vi "main.vi"(11 "Module Admin":refnum<class "Delacor_lib_QMH_Module Admin.lvclass">) -> ()   [LabVIEW 2020, in "G-AI Core.lvlib"]
doc: "This template is based off of the Queued Message Handler design pattern and the Queued Message Handler project template that ships with LabVIEW.\n\nThe main difference is that the queue is private to this module and communication between modules is performed via Broadcast and Request events.\n\nRequest events are wrapped in public API methods and are handled in the Event Handling Loop (EHL) of this VI. Any module can register for Broadcast events sent by this module. The EHL generates messages based on user interface actions.\n\nThe Message Handling Loop (MHL) processes messages generated by the EHL, or by other messages. The messages are string values, so new messages can be added easily to the Message Cases case structure in the MHL. Each message cluster can also provide an optional value for Message Data, which is a variant that can be converted to whatever message-specific data is required.\n_____\nBased on DQMH Dev Tools: Project Template 7.1.2.1547."
uses:
  G-AI Core.lvlib
  <vilib>/Delacor/Delacor QMH/Libraries/Module Admin_class/Delacor_lib_QMH_Module Admin.lvclass
  Module Data--cluster.ctl
  <vilib>/Delacor/Delacor QMH/Libraries/Message Queue_class/Delacor_lib_QMH_Message Queue.lvclass/Delacor_lib_QMH_Message Queue.ctl
  Stop Argument--cluster.ctl
  <vilib>/Delacor/Delacor QMH/Libraries/Module Admin_class/Delacor_lib_QMH_Module Admin.lvclass/Delacor_lib_QMH_Module Admin.ctl
  Store Reference Argument--cluster.ctl
  Store Reference (Reply Payload)--cluster.ctl
  Get Reference Argument--cluster.ctl
  Get Reference (Reply Payload)--cluster.ctl
  New VI Argument--cluster.ctl
  New VI (Reply Payload)--cluster.ctl
  Open VI Reference Argument--cluster.ctl
  Open VI Reference (Reply Payload)--cluster.ctl
  <vilib>/Utility/miscctls.llb/LVPointTypeDef.ctl
  <vilib>/Delacor/Delacor QMH/Libraries/Message Queue_class/Delacor_lib_QMH_Enqueue Message (Single).vi
  <vilib>/Delacor/Delacor QMH/Libraries/Module Admin_class/Delacor_lib_QMH_Get External Launch.vi
  <vilib>/Delacor/Delacor QMH/Libraries/Message Queue_class/Delacor_lib_QMH_Message Queue.lvclass
  <vilib>/jgoebel/LabVIEW MCP Server SDK/src/MCP Server/jg_mcp_MCP Server.lvlib
panel:
  out "Log":string
  out "error out":errorcluster
  out "Status":string
  in  "Simulate MHL Error":bool
  in  "Simulate EHL Error":bool
  # "Keep this VI open to make the G-AI MCP-Server reachable from your\nMCP Client (e.g. Claude Desktop).\nAdd MCP Server to mcp_config.json or claude_desktop_config.json"
  # "Server Name: G-AI\nServer Port: 36987\nServer URL: /mcp/server"
  # "https://github.com/JanGoebel/G-AI"
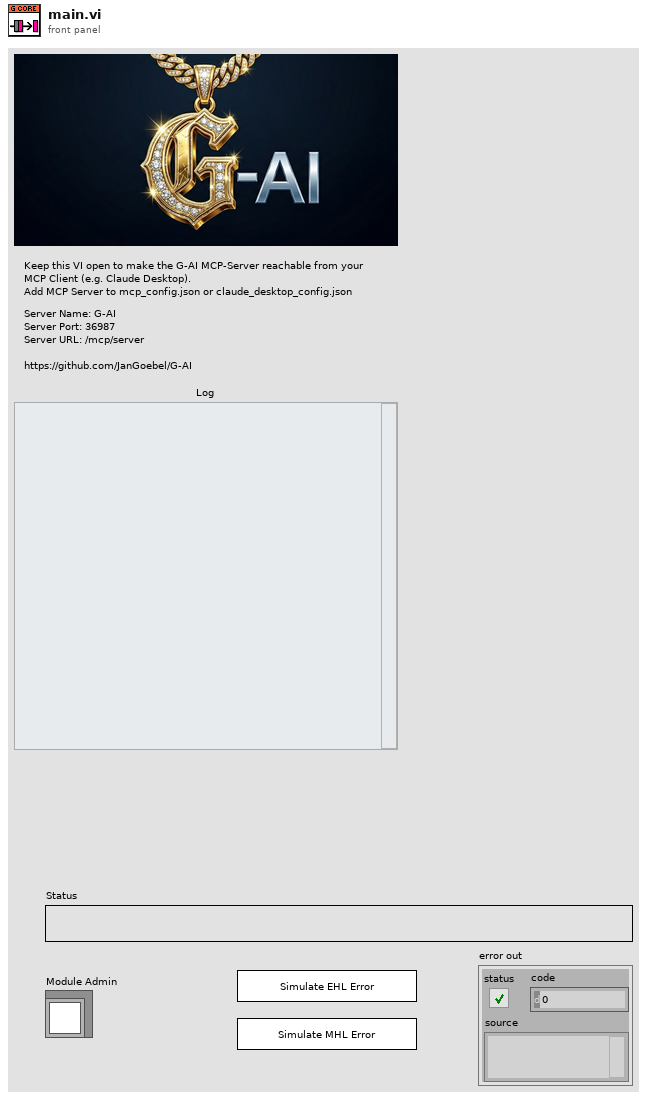
[diagram p1: front panel]
types:
  T1 = typedef "G-AI Core.lvlib/Module Data--cluster.ctl" = cluster{"Status":string, "LookupTable":variant, "last id":i32, "MCP reference":i32}
  T2 = typedef "G-AI Core.lvlib/Request Events--cluster.ctl" = cluster{"Stop Module":refnum<user-event>, "Show Panel":refnum<user-event>, "Hide Panel":refnum<user-event>, "Get Module Execution Status":refnum<user-event>, "Show Diagram":refnum<user-event>, "Store Reference":refnum<user-event>, "Get Reference":refnum<user-event>, "New VI":refnum<user-event>, "Open VI Reference":refnum<user-event>}
  T3 = typedef "jg_mcp_MCP Server.lvlib/jg_mcp_User Events.ctl" = cluster{"onError":refnum<user-event>, "onRpc":refnum<user-event>}
  T4 = enum32{"invalid lock state", "Not Locked", "Locked (No Password)", "Password-protected"}
  T5 = typedef "G-AI Core.lvlib/Stop Argument--cluster.ctl" = cluster{"Origin":string, "Exit via Stop Module Req?":bool, "Wait for Module to stop?":bool}
  T6 = typedef "G-AI Core.lvlib/Store Reference Argument--cluster.ctl" = cluster{"Reference":variant, "Wait Notifier":refnum<notifier>, "wait for reply":bool}
  T7 = typedef "G-AI Core.lvlib/Get Reference Argument--cluster.ctl" = cluster{"id":string, "Wait Notifier":refnum<notifier>, "wait for reply":bool}
  T8 = typedef "G-AI Core.lvlib/New VI Argument--cluster.ctl" = cluster{"Wait Notifier":refnum<notifier>, "wait for reply":bool}
  T9 = typedef "G-AI Core.lvlib/Open VI Reference Argument--cluster.ctl" = cluster{"VI Path":string, "options":i32, "password":string, "Wait Notifier":refnum<notifier>, "wait for reply":bool}
  T10 = typedef "LVPointTypeDef.ctl" = cluster{"Horizontal":i16, "Vertical":i16}
  T11 = enum32{"Invalid", "Standard", "Closed", "Hidden", "Minimized", "Maximized"}
  T12 = typedef "G-AI Core.lvlib/New VI (Reply Payload)--cluster.ctl" = cluster{"VI Refnum":refnum<vi>, "error":errorcluster}
  T13 = typedef "G-AI Core.lvlib/Open VI Reference (Reply Payload)--cluster.ctl" = cluster{"VI Refnum":refnum<vi>, "error":errorcluster}
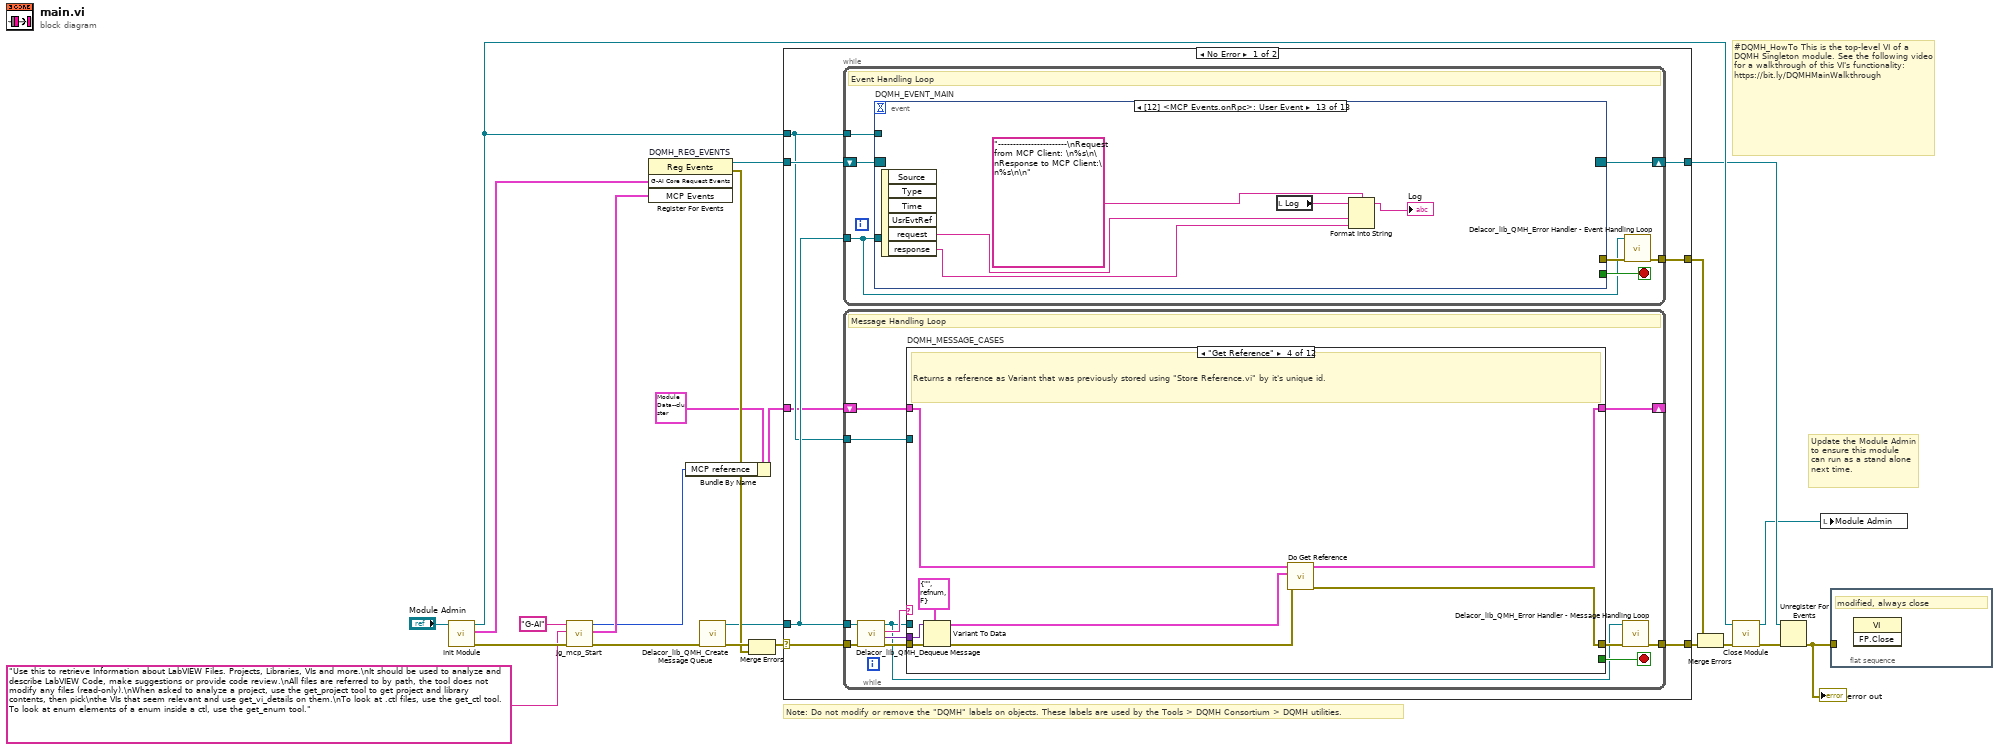
[diagram p0: block diagram]
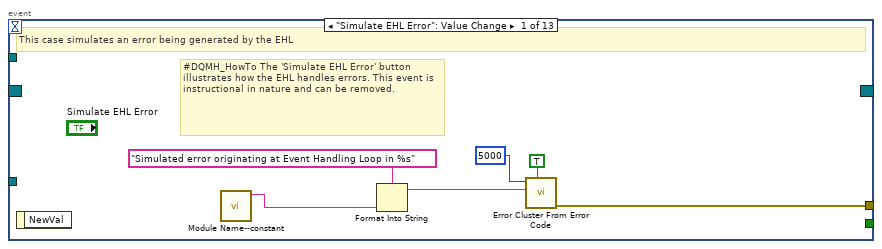
[diagram p2: hidden frame]
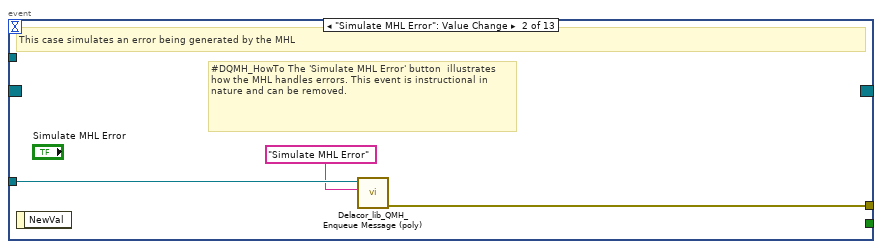
[diagram p3: hidden frame]
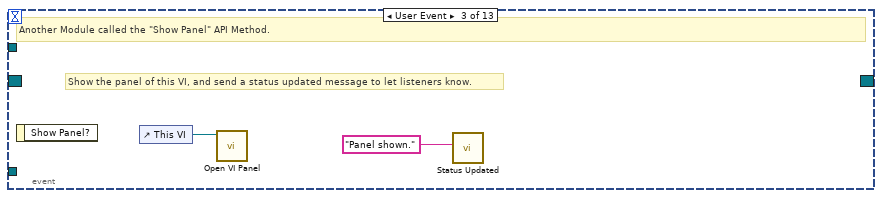
[diagram p4: hidden frame]
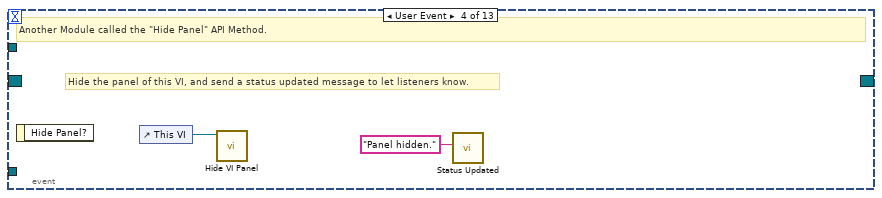
[diagram p5: hidden frame]
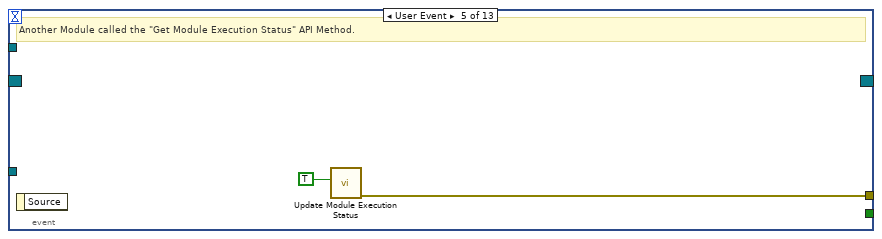
[diagram p6: hidden frame]
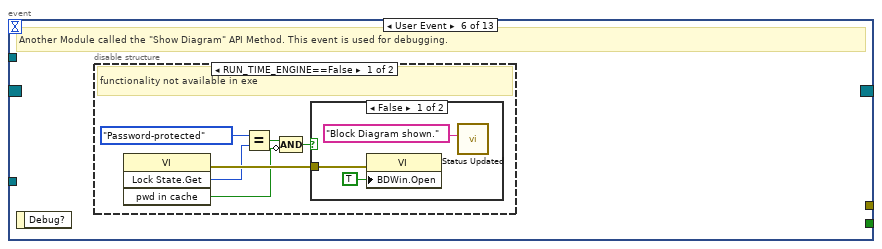
[diagram p7: hidden frame]
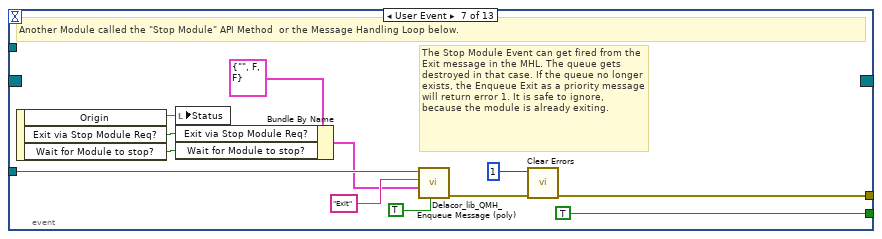
[diagram p10: hidden frame]
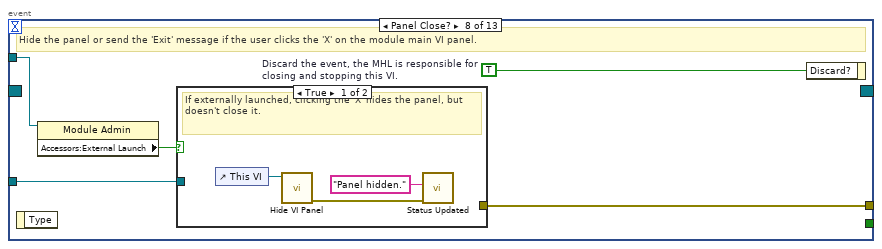
[diagram p11: hidden frame]
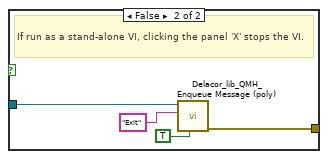
[diagram p12: hidden frame]
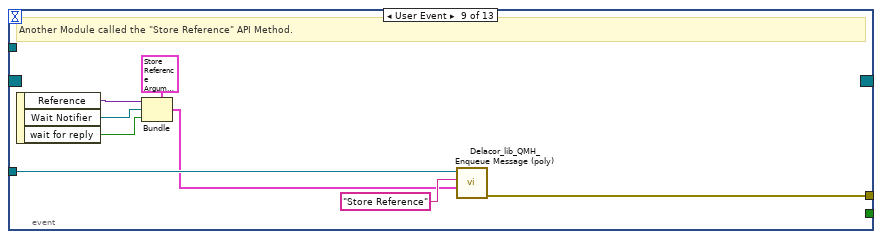
[diagram p13: hidden frame]
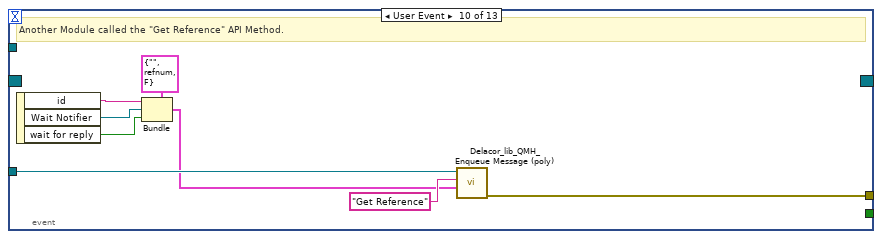
[diagram p14: hidden frame]
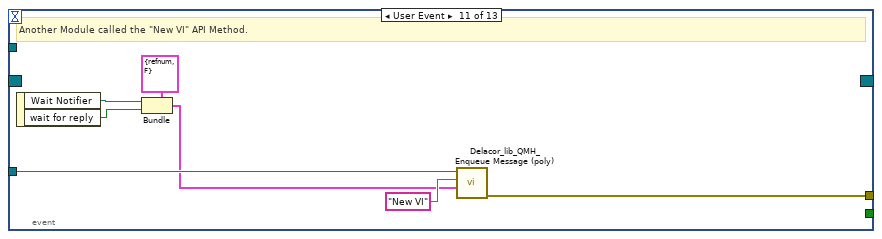
[diagram p15: hidden frame]
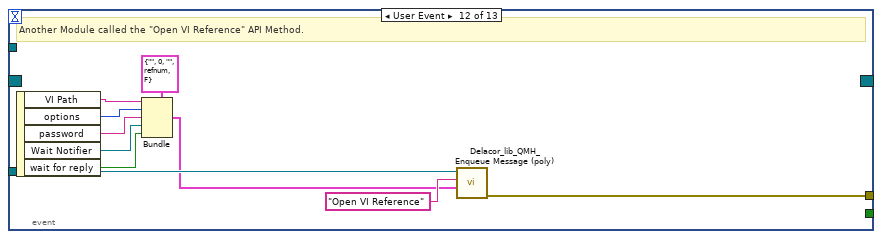
[diagram p16: hidden frame]
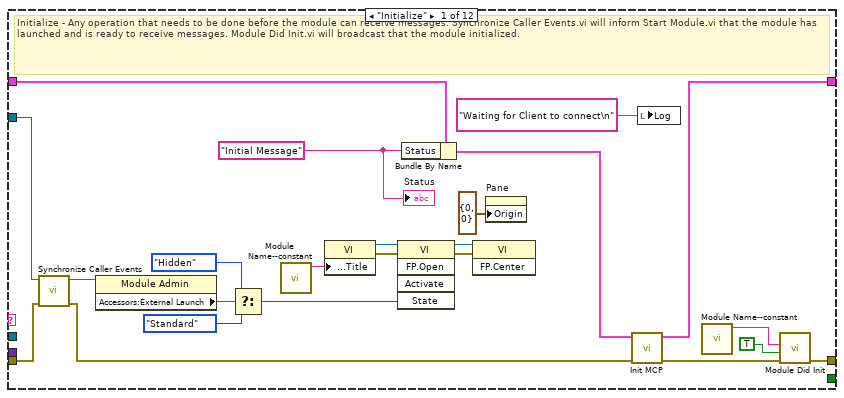
[diagram p17: hidden frame]
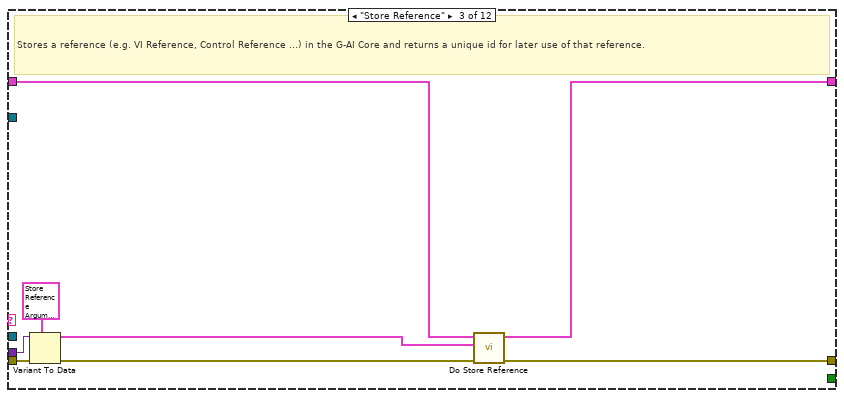
[diagram p19: hidden frame]
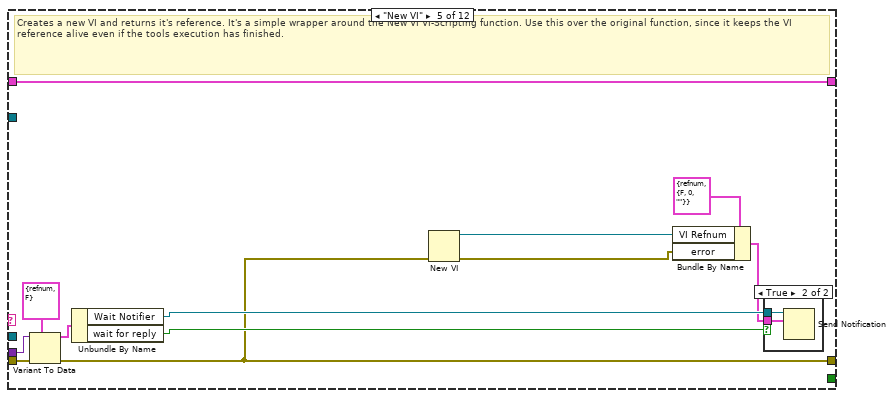
[diagram p20: hidden frame]
diagram:
  # "#DQMH_HowTo This is the top-level VI of a DQMH Singleton module. See the following video for a walkthrough of this VI's functionality: https://bit.ly/DQMHMainWalkthrough"
  # "Note: Do not modify or remove the \"DQMH\" labels on objects. These labels are used by the Tools > DQMH Consortium > DQMH utilities."
  # "Update the Module Admin to ensure this module can run as a stand alone next time."
  n1 = call "Init Module.vi"("Singleton Module Admin in"="Module Admin") -> ("error out"=w9:errorcluster, "G-AI Core Request Events"=w13:T2, "Singleton Module Admin out"=w16:refnum<class "Delacor_lib_QMH_Module Admin.lvclass">)  [unwired: 8 in]
  n2 = call <vilib>:"jg_mcp_Start.vi"("error in (no error)"=w9, "Description"="Use this to retrieve Information about LabVIEW Files. Projects, Libraries, VIs and more.\nIt should be used to analyze and describe LabVIEW Code, make suggestions or provide code review.\nAll files are referred to by path, the tool does not modify any files (read-only).\nWhen asked to analyze a project, use the get_project tool to get project and library contents, then pick\nthe VIs that seem relevant and use get_vi_details on them.\nTo look at .ctl files, use the get_ctl tool. To look at enum elements of a enum inside a ctl, use the get_enum tool.", "Name"="G-AI") -> ("error out"=w8:errorcluster, "MCP Events"=w5:T3, "server id out"=w2:i32)  [unwired: 6 in]
  n3 = register-events "DQMH_REG_EVENTS"(w13, w5) -> (reference out=w14:refnum<event-registration>, error out=w17:errorcluster)  [unwired: 2 in]
  n4 = Bundle By Name(cluster=T1 {"Status"="", "LookupTable"=variant, "last id"=0, "MCP reference"=0} ("Data Cluster"), "MCP reference"=w2) -> (w3:T1)
  n5 = call <vilib>:"Delacor_lib_QMH_Create Message Queue.vi"("error in"=w8) -> ("error out"=w19:errorcluster, "Message Queue"=w12:refnum<class "Delacor_lib_QMH_Message Queue.lvclass">)  [unwired: 9 in]
  n6 = Merge Errors(w19, w17) -> (w18:errorcluster)
  n7 = case shown="No Error" w18 {
    selector: w18 -> [w29 w274]
    tunnel: [w31 w273] -> w23
    tunnel: [w28 w272] -> w15
    tunnel: w14 -> [w27 w272]
    tunnel: w12 -> [w26 w267]
    tunnel: [w30 _] -> w21
    tunnel: w16 -> [w25 w268]
    tunnel: w3 -> [w24 _]
    frame No Error {
      n8 = while {
        tunnel: w26 -> [w32]
        shift-right: [w35] -> w28
        shift-left: w27 -> [w36]
        tunnel: [w37] -> w30
        tunnel: w25 -> [w33]
        stop <- w34 stop-if-true
        # "Event Handling Loop"
        n9 = event "DQMH_EVENT_MAIN" shown="[12] <MCP Events.onRpc>: User Event" {
          selector: w36 -> [_ _ _ _ _ _ _ _ _ _ _ _ _]
          dyn-events: [_ _ _ _ _ _ _ _ _ _ _ _ _] -> w35
          timeout: _ -> [_ _ _ _ _ _ _ _ _ _ _ _ _]
          tunnel: [_ _ _ _ _ _ TRUE ("Discard?") _ _ _ _ _ _] -> w34
          tunnel: w32 -> [_ w46 _ _ _ _ w70 w77 w94 w102 w109 w119 _]
          tunnel: [w44 w47 _ _ w53 _ w73 w79 w87 w95 w103 w110 _] -> w38
          tunnel: w33 -> [_ _ _ _ _ _ _ w76 _ _ _ _ _]
          event "Simulate EHL Error": Value Change {
            # "#DQMH_HowTo The 'Simulate EHL Error' button  illustrates how the EHL handles errors. This event is instructional in nature and can be removed."
            # "This case simulates an error being generated by the EHL"
            n10 = event-data() -> ()  [unwired: 1 in, 1 out]
            n11 = call "Module Name--constant.vi"() -> ("Module Name"=w41:string)  [unwired: 11 in]
            n12 = Format Into String(format string="Simulated error originating at Event Handling Loop in %s", w41) -> (resulting string=w42:string)  [unwired: 2 in, 1 out]
            n13 = call <vilib>:"Error Cluster From Error Code.vi"("show call chain? (False)"=TRUE, "error message (\"\")"=w42, "error code (0)"=5000) -> ("error out"=w44:errorcluster)  [unwired: 6 in]
          }
          event "Simulate MHL Error": Value Change {
            # "#DQMH_HowTo The 'Simulate MHL Error' button  illustrates how the MHL handles errors. This event is instructional in nature and can be removed."
            # "This case simulates an error being generated by the MHL"
            n14 = event-data() -> ()  [unwired: 1 in, 1 out]
            n15 = call-poly <vilib>:"Delacor_lib_QMH_Enqueue Message (poly).vi"("Message"="Simulate MHL Error", "Message Queue in"=w46) -> ("error out"=w47:errorcluster)  [unwired: 8 in, 1 out]
          }
          event User Event {
            # "Show the panel of this VI, and send a status updated message to let listeners know."
            # "Another Module called the \"Show Panel\" API Method."
            n16 = event-data() -> ()  [unwired: 1 in, 1 out]
            n17 = control-ref of="This VI"() -> (w49:refnum<vi>)
            n18 = call "Open VI Panel.vi"("VI"=w49) -> ()  [unwired: 10 in, 1 out]
            n19 = call "Status Updated.vi"("Status"="Panel shown." ("format string")) -> ()  [unwired: 10 in, 1 out]
          }
          event User Event {
            # "Hide the panel of this VI, and send a status updated message to let listeners know."
            # "Another Module called the \"Hide Panel\" API Method."
            n20 = event-data() -> ()  [unwired: 1 in, 1 out]
            n21 = control-ref of="This VI"() -> (w51:refnum<vi>)
            n22 = call "Hide VI Panel.vi"("VI"=w51) -> ()  [unwired: 10 in, 1 out]
            n23 = call "Status Updated.vi"("Status"="Panel hidden." ("format string")) -> ()  [unwired: 10 in, 1 out]
          }
          event User Event {
            # "Another Module called the \"Get Module Execution Status\" API Method."
            n24 = event-data() -> ()  [unwired: 1 in, 1 out]
            n25 = call "Update Module Execution Status.vi"("Running?"=TRUE) -> ("error out"=w53:errorcluster)  [unwired: 10 in]
          }
          event User Event {
            # "Another Module called the \"Show Diagram\" API Method. This event is used for debugging."
            n26 = event-data() -> ()  [unwired: 1 in, 1 out]
            n27 = disable-structure shown="RUN_TIME_ENGINE==False" {
              frame condition #0 (active) {
                # "functionality not available in exe"
                n28 = invoke on="Invoke Node" class="VI" method="Lock State.Get"() -> (error out=w59:errorcluster, "Get Lock State"=w58:T4, "pwd in cache"=w55:bool)  [unwired: 4 in, 1 out]
                n29 = Equal?(x=T4."Password-protected", y=w58) -> (x = y?=w56:bool)
                n30 = Compound Arithmetic op=AND(w56, invert w55) -> (w54:bool)
                n31 = case shown="False" w54 {
                  tunnel: w59 -> [w62 _]
                  frame False {
                    n32 = property on="Property Node" class="VI"(error in=w62, "BDWin.Open"=TRUE ("Block Diagram Window:Open")) -> ()  [unwired: 1 in, 2 out]
                    n33 = call "Status Updated.vi"("Status"="Block Diagram shown." ("format string")) -> ()  [unwired: 10 in, 1 out]
                  }
                  frame True {
                    # "Password-protected VI, and the password is not in the cache. Do not show the diagram."
                  }
                }
              }
              frame condition #1 {
              }
            }
          }
          event User Event {
            # "The Stop Module Event can get fired from the Exit message in the MHL. The queue gets destroyed in that case. If the queue no longer exists, the Enqueue Exit as a priority message will return error 1. It is safe to ignore, because the module is already exiting."
            # "Another Module called the \"Stop Module\" API Method  or the Message Handling Loop below."
            n34 = event-data() -> ("Origin"=w69:string, "Exit via Stop Module Req?"=w65:bool, "Wait for Module to stop?"=w64:bool)  [unwired: 1 in]
            n35 = local write "Status"(w69) -> ()
            n36 = Bundle By Name(cluster=T5 {"Origin"="", "Exit via Stop Module Req?"=FALSE, "Wait for Module to stop?"=FALSE} ("Stop Argument"), "Exit via Stop Module Req?"=w65, "Wait for Module to stop?"=w64) -> (w63:T5)
            n37 = call-poly <vilib>:"Delacor_lib_QMH_Enqueue Message (poly).vi"("Priority Message? (F)"=TRUE, "Message Data"=w63, "Message"="Exit", "Message Queue in"=w70) -> ("error out"=w74:errorcluster)  [unwired: 6 in, 1 out]
            n38 = call <vilib>:"Clear Errors.vi"("error in (no error)"=w74, "specific error code to clear (0: all)"=1) -> ("error out"=w73:errorcluster)  [unwired: 4 in, 1 out]
          }
          event Panel Close? {
            w78 = TRUE  # Discard the event, the MHL is responsible for closing and stopping this VI.
            # "Hide the panel or send the 'Exit' message if the user clicks the 'X' on the module main VI panel."
            n39 = event-data() -> ()  [unwired: 1 in, 1 out]
            n40 = property on="Property Node" class="Module Admin"(reference=w76) -> ("Accessors:External Launch"=w75:bool)  [unwired: 1 in, 2 out]
            n41 = case shown="True" w75 {
              tunnel: w77 -> [_ w85]
              tunnel: [_ w86] -> w79
              frame True {
                # "If externally launched, clicking the 'X' hides the panel, but doesn't close it."
                n42 = control-ref of="This VI"() -> (w82:refnum<vi>)
                n43 = call "Hide VI Panel.vi"("VI"=w82) -> ("error out"=w80:errorcluster)  [unwired: 10 in]
                n44 = call "Status Updated.vi"("error in"=w80, "Status"="Panel hidden." ("format string")) -> ()  [unwired: 9 in, 1 out]
              }
              frame False {
                # "If run as a stand-alone VI, clicking the panel 'X' stops the VI."
                n45 = call-poly <vilib>:"Delacor_lib_QMH_Enqueue Message (poly).vi"("Priority Message? (F)"=TRUE, "Message"="Exit", "Message Queue in"=w85) -> ("error out"=w86:errorcluster)  [unwired: 7 in, 1 out]
              }
            }
            n46 = event-data ("Event Filter Node")("Discard?"=w78) -> ()  [unwired: 1 in, 1 out]
          }
          event User Event {
            # "Another Module called the \"Store Reference\" API Method."
            n47 = event-data() -> ("Reference"=w90:variant, "Wait Notifier"=w89:refnum<notifier>, "wait for reply"=w88:bool)  [unwired: 1 in]
            n48 = Bundle(cluster=T6 {"Reference"=variant, "Wait Notifier"=refnum, "wait for reply"=FALSE} ("Store Reference Argument"), "Reference"=w90, "Wait Notifier"=w89, "wait for reply"=w88) -> (w91:T6)
            n49 = call-poly <vilib>:"Delacor_lib_QMH_Enqueue Message (poly).vi"("Message Data"=w91, "Message"="Store Reference", "Message Queue in"=w94) -> ("error out"=w87:errorcluster)  [unwired: 7 in, 1 out]
          }
          event User Event {
            # "Another Module called the \"Get Reference\" API Method."
            n50 = event-data() -> ("id"=w98:string, "Wait Notifier"=w97:refnum<notifier>, "wait for reply"=w96:bool)  [unwired: 1 in]
            n51 = Bundle(cluster=T7 {"id"="", "Wait Notifier"=refnum, "wait for reply"=FALSE} ("Get Reference Argument"), "id"=w98, "Wait Notifier"=w97, "wait for reply"=w96) -> (w99:T7)
            n52 = call-poly <vilib>:"Delacor_lib_QMH_Enqueue Message (poly).vi"("Message Data"=w99, "Message"="Get Reference", "Message Queue in"=w102) -> ("error out"=w95:errorcluster)  [unwired: 7 in, 1 out]
          }
          event User Event {
            # "Another Module called the \"New VI\" API Method."
            n53 = event-data() -> ("Wait Notifier"=w105:refnum<notifier>, "wait for reply"=w104:bool)  [unwired: 1 in]
            n54 = Bundle(cluster=T8 {"Wait Notifier"=refnum, "wait for reply"=FALSE} ("New VI Argument"), "Wait Notifier"=w105, "wait for reply"=w104) -> (w106:T8)
            n55 = call-poly <vilib>:"Delacor_lib_QMH_Enqueue Message (poly).vi"("Message Data"=w106, "Message"="New VI", "Message Queue in"=w109) -> ("error out"=w103:errorcluster)  [unwired: 7 in, 1 out]
          }
          event User Event {
            # "Another Module called the \"Open VI Reference\" API Method."
            n56 = event-data() -> ("VI Path"=w115:string, "options"=w114:i32, "password"=w113:string, "Wait Notifier"=w112:refnum<notifier>, "wait for reply"=w111:bool)  [unwired: 1 in]
            n57 = Bundle(cluster=T9 {"VI Path"="", "options"=0, "password"="", "Wait Notifier"=refnum, "wait for reply"=FALSE} ("Open VI Reference Argument"), "VI Path"=w115, "options"=w114, "password"=w113, "Wait Notifier"=w112, "wait for reply"=w111) -> (w116:T9)
            n58 = call-poly <vilib>:"Delacor_lib_QMH_Enqueue Message (poly).vi"("Message Data"=w116, "Message"="Open VI Reference", "Message Queue in"=w119) -> ("error out"=w110:errorcluster)  [unwired: 7 in, 1 out]
          }
          event User Event {
            n59 = event-data() -> ("request"=w123:string, "response"=w122:string)  [unwired: 1 in, 4 out]
            n60 = local read "Log"() -> (w120:string)
            n61 = Format Into String(format string="-----------------------\nRequest from MCP Client: \n%s\n\nResponse to MCP Client:\n%s\n\n", initial string=w120, w123, w122) -> (resulting string=→"Log":string)  [unwired: 1 in, 1 out]
          }
        }
        n62 = call-dynamic "Delacor_lib_QMH_Error Handler - Event Handling Loop.vi"("error in"=w38, "Message Queue in"=w32) -> ("dup error in"=w37:errorcluster)  [unwired: 8 in, 1 out]
      }
      n63 = while {
        tunnel: w26 -> [w125]
        shift-right: [w133] -> _
        shift-left: w24 -> [w134]
        tunnel: w29 -> [w136]
        tunnel: [w128] -> w31
        tunnel: w25 -> [w129]
        stop <- w132 stop-if-true
        # "Message Handling Loop"
        n64 = call-dynamic "Delacor_lib_QMH_Dequeue Message.vi"("error in"=w136, "Message Queue in"=w125) -> ("error out"=w135:errorcluster, "Message Data"=w130:variant, "Message"=w131:string, "Message Queue out"=w126:refnum<class "Delacor_lib_QMH_Message Queue.lvclass">)  [unwired: 6 in]
        n65 = case "DQMH_MESSAGE_CASES" shown="\"Get Reference\"" w131 {
          selector: w131 -> [_ _ _ _ _ _ _ _ _ _ _ w262]
          tunnel: w126 -> [_ _ _ _ _ _ _ _ _ w226 w251 _]
          tunnel: w135 -> [w157 w161 w169 w177 w189 w206 w211 w213 w222 w233 w256 w265]
          tunnel: [w155 w161 w163 w171 w179 w204 w210 w213 w221 w229 w252 w266] -> w127
          tunnel: w134 -> [w146 w160 w168 w176 w188 w205 w209 w212 w219 w228 w241 w263]
          tunnel: [w139 w160 w162 w170 w188 w205 w209 w212 w219 w228 w241 w263] -> w133
          tunnel: [_ _ _ _ _ _ _ _ _ _ w250 _] -> w132
          tunnel: w130 -> [_ _ w166 w174 w187 w203 _ _ _ w227 w249 _]
          tunnel: w129 -> [w147 _ _ _ _ _ _ _ _ w225 w244 _]
          frame "Initialize" {
            w141 = "Initial Message" ("Initial Message")
            # "Initialize - Any operation that needs to be done before the module can receive messages. Synchronize Caller Events.vi will inform Start Module.vi that the module has launched and is ready to receive messages. Module Did Init.vi will broadcast that the module initialized."
            n66 = call "Synchronize Caller Events.vi"("error in"=w157, "Singleton Module Admin in"=w147) -> ("error out"=w156:errorcluster, "Singleton Module Admin out"=w142:refnum<class "Delacor_lib_QMH_Module Admin.lvclass">)  [unwired: 8 in]
            n67 = property on="Property Node" class="Module Admin"(reference=w142) -> ("Accessors:External Launch"=w151:bool)  [unwired: 1 in, 2 out]
            n68 = Select(t=T11."Hidden" ("State"), s=w151, f=T11."Standard" ("State")) -> (s? t:f=w148:T11)
            n69 = call "Module Name--constant.vi"() -> ("Module Name"=w154:string)  [unwired: 11 in]
            n70 = property on="Property Node" class="VI"("Front Panel.Title"=w154) -> (reference out=w153:refnum<vi>, error out=w159:errorcluster)  [unwired: 2 in]
            n71 = invoke on="Invoke Node" class="VI" method="FP.Open"(reference=w153, error in=w159, "State"=w148) -> (reference out=w152:refnum<vi>, error out=w158:errorcluster)  [unwired: 2 in, 3 out]
            n72 = Bundle By Name(cluster=w146, "Status"=w141) -> (w145:T1)
            n73 = invoke on="Invoke Node" class="VI" method="FP.Center"(reference=w152, error in=w158) -> ()  [unwired: 1 in, 3 out]
            n74 = property on="Pane" class="Pane"("Origin"=T10 {"Horizontal"=0, "Vertical"=0}) -> ()  [unwired: 2 in, 2 out]
            n75 = call "Init MCP.vi"("error in (no error)"=w156, "Data Cluster in"=w145) -> ("error out"=w138:errorcluster, "Data Cluster out"=w139:T1)  [unwired: 8 in]
            n76 = local write "Log"("Waiting for Client to connect\n") -> ()
            n77 = call "Module Name--constant.vi"() -> ("Module Name"=w143:string)  [unwired: 11 in]
            n78 = call "Module Did Init.vi"("error in"=w138, "Initialized?"=TRUE, "Origin"=w143) -> ("error out"=w155:errorcluster)  [unwired: 8 in]
            "Status" <- w141
          }
          frame "---Module Specific---" {
            # "Separator -- The following cases handle messages specific to this Module."
          }
          frame "Store Reference" {
            # "Stores a reference (e.g. VI Reference, Control Reference ...) in the G-AI Core and returns a unique id for later use of that reference."
            n79 = Variant To Data(error in=w169, type=T6 {"Reference"=variant, "Wait Notifier"=refnum, "wait for reply"=FALSE} ("Store Reference Argument"), Variant=w166) -> (data=w164:T6, error out=w167:errorcluster)
            n80 = call "Do Store Reference.vi"("error in (no error)"=w167, "Store Reference Argument"=w164, "Data Cluster in"=w168) -> ("error out"=w163:errorcluster, "Data Cluster out"=w162:T1)  [unwired: 7 in]
          }
          frame "Get Reference" {
            # "Returns a reference as Variant that was previously stored using \"Store Reference.vi\" by it's unique id."
            n81 = Variant To Data(error in=w177, type=T7 {"id"="", "Wait Notifier"=refnum, "wait for reply"=FALSE} ("Get Reference Argument"), Variant=w174) -> (data=w172:T7, error out=w175:errorcluster)
            n82 = call "Do Get Reference.vi"("error in (no error)"=w175, "Get Reference Argument"=w172, "Data Cluster in"=w176) -> ("error out"=w171:errorcluster, "Data Cluster out"=w170:T1)  [unwired: 7 in]
          }
          frame "New VI" {
            # "Creates a new VI and returns it's reference. It's a simple wrapper around the New VI VI-Scripting function. Use this over the original function, since it keeps the VI reference alive even if the tools execution has finished."
            n83 = Variant To Data(error in=w189, type=T8 {"Wait Notifier"=refnum, "wait for reply"=FALSE} ("New VI Argument"), Variant=w187) -> (data=w185:T8, error out=w179:errorcluster)
            n84 = Unbundle By Name(w185) -> ("Wait Notifier"=w184:refnum<notifier>, "wait for reply"=w183:bool)
            n85 = New VI(8:w179) -> (0:w178:errorcluster, 3:w180:refnum<vi>)  [unwired: 6 in]
            n86 = Bundle By Name(cluster=T12 {"VI Refnum"=refnum, "error"={"status"=FALSE, "code"=0, "source"=""}} ("New VI (Reply Payload)"), "VI Refnum"=w180, "error"=w178) -> (w182:T12)
            n87 = case "DQMH_FIRE_NOTIFIER" shown="True" w183 {
              tunnel: w184 -> [_ w191]
              tunnel: w182 -> [_ w190]
              frame False {
              }
              frame True {
                n88 = Send Notification(notification=w190, notifier=w191) -> ()  [unwired: 1 in, 2 out]
              }
            }
          }
          frame "Open VI Reference" {
            # "Wrapper for \"Open VI Reference\" function. Use this instead of the original function to make sure the VI Reference stays alive even if the tool finishes execution."
            n89 = Variant To Data(error in=w206, type=T9 {"VI Path"="", "options"=0, "password"="", "Wait Notifier"=refnum, "wait for reply"=FALSE} ("Open VI Reference Argument"), Variant=w203) -> (data=w201:T9, error out=w204:errorcluster)
            n90 = Unbundle By Name(w201) -> ("VI Path"=w194:string, "options"=w193:i32, "password"=w192:string, "Wait Notifier"=w200:refnum<notifier>, "wait for reply"=w199:bool)
            n91 = Open VI Reference(vi path=w194, options=w193, password ("")=w192) -> (vi reference=w195:refnum<vi>, error out=w196:errorcluster)  [unwired: 3 in]
            n92 = Bundle By Name(cluster=T13 {"VI Refnum"=refnum, "error"={"status"=FALSE, "code"=0, "source"=""}} ("Open VI Reference (Reply Payload)"), "VI Refnum"=w195, "error"=w196) -> (w198:T13)
            n93 = case "DQMH_FIRE_NOTIFIER" shown="True" w199 {
              tunnel: w200 -> [_ w208]
              tunnel: w198 -> [_ w207]
              frame False {
              }
              frame True {
                n94 = Send Notification(notification=w207, notifier=w208) -> ()  [unwired: 1 in, 2 out]
              }
            }
          }
          frame "---Copy This Frame---" {
            # "Duplicate this frame when creating new messages.  Change this comment in the duplicated frame to describe this message."
            n95 = Merge Errors(w211) -> (w210:errorcluster)
          }
          frame "---Exit and Error Handling---" {
            # "Separator - The following cases handle errors and exit messages."
          }
          frame "Simulate MHL Error" {
            # "#DQMH_HowTo The 'Simulate MHL Error' button  illustrates how the MHL handles errors. This event is instructional in nature and can be removed."
            # "Simulate an error occurring at the MHL"
            n96 = call "Module Name--constant.vi"() -> ("Module Name"=w215:string)  [unwired: 11 in]
            n97 = Format Into String(format string="Simulated error originating at Message Handling Loop in %s", w215) -> (resulting string=w216:string)  [unwired: 2 in, 1 out]
            n98 = call <vilib>:"Error Cluster From Error Code.vi"("show call chain? (False)"=TRUE, "error message (\"\")"=w216, "error code (0)"=5001) -> ("error out"=w220:errorcluster)  [unwired: 6 in]
            n99 = Merge Errors(w222, w220) -> (w221:errorcluster)
          }
          frame "Error" {
            # "#DQMH_CodeRecommended - If the module is running in standalone mode (External Launch = FALSE), this code will pop up an error dialog and call the 'Exit' message if an error occurs. Add more fine-grained error management here."
            # "Error - Check the error message data and respond accordingly. This message is sent by the \"Error Handler\" VIs at the end of each loop in this application."
            n100 = property on="Property Node" class="Module Admin"(reference=w225) -> ("Accessors:External Launch"=w224:bool)  [unwired: 1 in, 2 out]
            n101 = Variant To Data(error in=w233, type=errorcluster {"status"=FALSE, "code"=0, "source"=""} ("error constant"), Variant=w227) -> (data=w223:errorcluster, error out=w231:errorcluster)
            n102 = local write "error out"(w223) -> ()
            n103 = call "Error Reported.vi"("Error"=w223) -> ()  [unwired: 10 in, 1 out]
            n104 = case shown="False" w224 {
              tunnel: [w238 _] -> w230
              tunnel: w226 -> [w236 _]
              tunnel: w223 -> [w237 _]
              frame False {
                n105 = disable-structure shown="Default" {
                  disable-tunnel: w237 -> [w239 _]
                  frame condition #0 (active) {
                    # "If the module is running standalone, then pop up an error dialog and call the \"Exit\" message."
                    n106 = call <vilib>:"Simple Error Handler.vi"("error in (no error)"=w239) -> ()  [unwired: 4 in, 5 out]
                  }
                  frame condition #1 {
                    # "To prevent the Simple Error Handler VI from being loaded (e.g. when deploying to a Real-Time target), add the Conditional Disable Symbol \"DQMH_Disable_SEH\" to your project and set it to TRUE."
                  }
                }
                n107 = call-poly <vilib>:"Delacor_lib_QMH_Enqueue Message (poly).vi"("Priority Message? (F)"=TRUE, "Message"="Exit", "Message Queue in"=w236) -> ("error out"=w238:errorcluster)  [unwired: 7 in, 1 out]
              }
              frame True {
                # "If the module was launched externally, calling the Error Reported broadcast VI is the only action performed by the \"Error\" message. The module's caller can then process the error appropriately."
              }
            }
            n108 = Merge Errors(w231, w230) -> (w229:errorcluster)
          }
          frame "Exit" {
            w248 = 91  # 91: not all Exit messages will have an argument
            w250 = TRUE  # Stop the VI
            # "Release the message queue reference"
            # "Exit - Exit the application."
            n109 = Variant To Data(error in=w256, type=T5 {"Origin"="", "Exit via Stop Module Req?"=FALSE, "Wait for Module to stop?"=FALSE} ("Stop Argument"), Variant=w249) -> (data=w246:T5, error out=w254:errorcluster)
            n110 = call <vilib>:"Clear Errors.vi"("error in (no error)"=w254, "specific error code to clear (0: all)"=w248) -> ("error out"=w255:errorcluster)  [unwired: 4 in, 1 out]
            n111 = control-ref of="This VI"() -> (w245:refnum<vi>)
            n112 = call-dynamic "Delacor_lib_QMH_Release Message Queue.vi"("error in"=w255, "Message Queue"=w251) -> ("error out"=w243:errorcluster)  [unwired: 9 in]
            n113 = call "Handle Exit.vi"("Stop Argument"=w246, "Admin in"=w244, "VI reference"=w245) -> ("error out"=w253:errorcluster)  [unwired: 7 in, 1 out]
            n114 = Unbundle By Name(w241) -> ("MCP reference"=w240:i32)
            n115 = call <vilib>:"jg_mcp_Stop.vi"("error in (no error)"=w243, "id"=w240) -> ("error out"=w242:errorcluster)  [unwired: 9 in]
            n116 = Merge Errors(w242, w253) -> (w252:errorcluster)
            n117 = call "Error Reported.vi"("Error"=w252) -> ()  [unwired: 10 in, 1 out]
          }
          frame Default {
            # "'Default' case only runs if there is a message that isn't defined in any of the other cases.  Output a programming error."
            n118 = call "Module Name--constant.vi"() -> ("Module Name"=w261:string)  [unwired: 11 in]
            n119 = Format Into String(format string="The invalid message string \"%s\" was received in the Message Handling Loop for module \"%s\".", w262, w261) -> (resulting string=w257:string)  [unwired: 2 in, 1 out]
            n120 = call <vilib>:"Error Cluster From Error Code.vi"("show call chain? (False)"=TRUE, "error message (\"\")"=w257, "error code (0)"=1) -> ("error out"=w264:errorcluster)  [unwired: 6 in]
            n121 = Merge Errors(w265, w264) -> (w266:errorcluster)
          }
        }
        n122 = call-dynamic "Delacor_lib_QMH_Error Handler - Message Handling Loop.vi"("error in"=w127, "Message Queue in"=w126) -> ("dup error in"=w128:errorcluster)  [unwired: 8 in, 1 out]
      }
    }
    frame Error {
      # "Synchronize Caller Events.vi will inform Start Module.vi that the module has launched and will let the code calling Start Module.vi register for broadcasts and would permit the caller receive the broadcast that an error occurred at launch time."
      n123 = call-dynamic "Delacor_lib_QMH_Release Message Queue.vi"("error in"=w274, "Message Queue"=w267) -> ("error out"=w273:errorcluster)  [unwired: 9 in]
      n124 = call "Synchronize Caller Events.vi"("Singleton Module Admin in"=w268) -> ("error out"=w275:errorcluster)  [unwired: 9 in, 1 out]
      n125 = call "Module Name--constant.vi"() -> ("Module Name"=w271:string)  [unwired: 11 in]
      n126 = Format Into String(format string="An error occurred during initialization. %s is no longer running.", w271) -> (resulting string=w269:string)  [unwired: 2 in, 1 out]
      n127 = Merge Errors(w273, w275) -> (w276:errorcluster)
      n128 = call "Error Reported.vi"("Additional Information"=w269, "Error"=w276) -> ()  [unwired: 9 in, 1 out]
    }
  }
  n129 = Merge Errors(w21, w23) -> (w20:errorcluster)
  n130 = call "Close Module.vi"("error in"=w20, "Module Admin in"=w16) -> ("error out"=w22:errorcluster, "Module Admin out"=w10:refnum<class "Delacor_lib_QMH_Module Admin.lvclass">)  [unwired: 7 in, 1 out]
  n131 = Unregister For Events(event registration refnum=w15, error in=w22) -> (error out=w1:errorcluster)
  "error out" <- w1
  n132 = local write "Module Admin"(w10) -> ()
  n133 = flat-sequence {
    tunnel: w1 -> [_]
    frame #0 {
      # "modified, always close"
      n134 = invoke on="Invoke Node" class="VI" method="FP.Close"() -> ()  [unwired: 3 in, 3 out]
    }
  }
